vi "Simple Generate 1.vi"(8 "Error In":errorcluster) -> (0 "Error Out":errorcluster)   [LabVIEW 2014, in "LabVIEW Universal Transcriptor AD9850.lvlib"]
uses:
  LabVIEW Universal Transcriptor AD9850.lvlib
  AD9850.lvclass
panel:
  in  "w_clk":i32=8
  in  "fq_ud":i32=9
  in  "data":i32=10
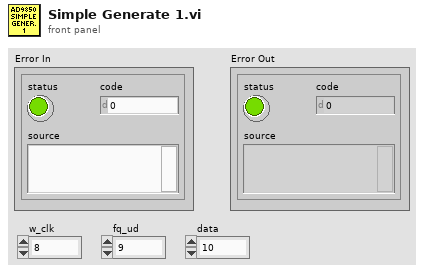
[diagram p1: front panel]
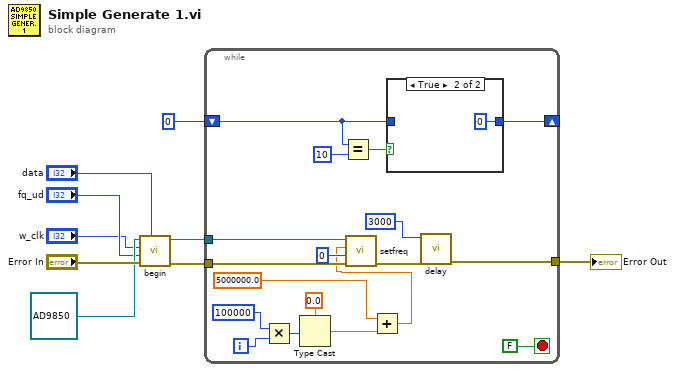
[diagram p0: block diagram]
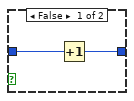
[diagram p2: hidden frame]
diagram:
  n1 = call-dynamic "begin.vi"("data"="data", "error in (no error)"="Error In", "fq_ud"="fq_ud", "w_clk"="w_clk", "AD9850 in"=refnum<class "AD9850.lvclass"> refnum) -> ("error out"=w3:errorcluster, "AD9850 out"=w2:refnum<class "AD9850.lvclass">)  [unwired: 5 in]
  n2 = while {
    shift-right: [w24] -> _
    shift-left: 0 -> [w26]
    tunnel: w3 -> [w21]
    tunnel: w2 -> [w20]
    tunnel: [w14] -> w1
    i -> [w23]
    stop <- FALSE stop-if-true
    n3 = Multiply(x=100000, y=w23) -> (x*y=w18:i32)
    n4 = Type Cast(type=0.0, x=w18) -> (*(type *) &x=w13:dbl)
    n5 = Equal?(x=w26, y=10) -> (x = y?=w27:bool)
    n6 = Add(x=5000000.0, y=w13) -> (x+y=w11:dbl)
    n7 = call-dynamic "setfreq.vi"("error in (no error)"=w21, "phase"=u8 0, "frequency"=w11, "AD9850 in"=w20) -> ("error out"=w16:errorcluster)  [unwired: 6 in, 1 out]
    n8 = case shown="True" w27 {
      tunnel: w26 -> [w29 _]
      tunnel: [w28 0] -> w24
      frame False {
        n9 = Increment(x=w29) -> (x+1=w28:i32)
      }
      frame True {
      }
    }
    n10 = call <vilib>:"delay.vi"("Error In"=w16, "time (ms)"=3000) -> ("Error Out"=w14:errorcluster)  [unwired: 9 in]
  }
  "Error Out" <- w1
